vi "Save Image.vi"(8 "error in (no error)":errorcluster, 10 "Screen Shot Path":path, 11 "VISA resource name":refnum<visa-resource-name>) -> (0 "error out":errorcluster, 3 "VISA resource name out":refnum<visa-resource-name>)   [LabVIEW 2018, in "DPO4104.lvlib" / "DPO4104.lvclass"]
doc: "This VI sends the command to save a screen shot to the location specified in the input path. Tested file extensions: .png, .bmp, .tiff, .jpg, .jpeg."
uses:
  DPO4104.lvclass
  <instrlib>/Tektronix DPO MSO 2000 4000 Series/Tektronix DPO MSO 2000 4000 Series.lvlib
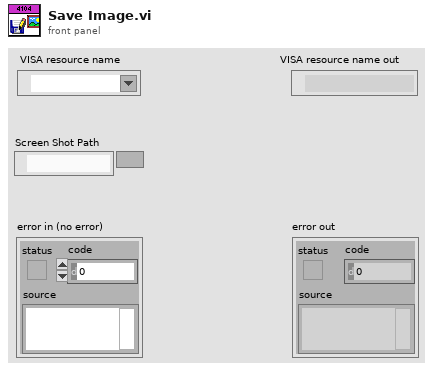
[diagram p1: front panel]
types:
  T1 = enum16{"open", "replace", "create", "open or create", "replace or create", "replace or create with confirmation"}
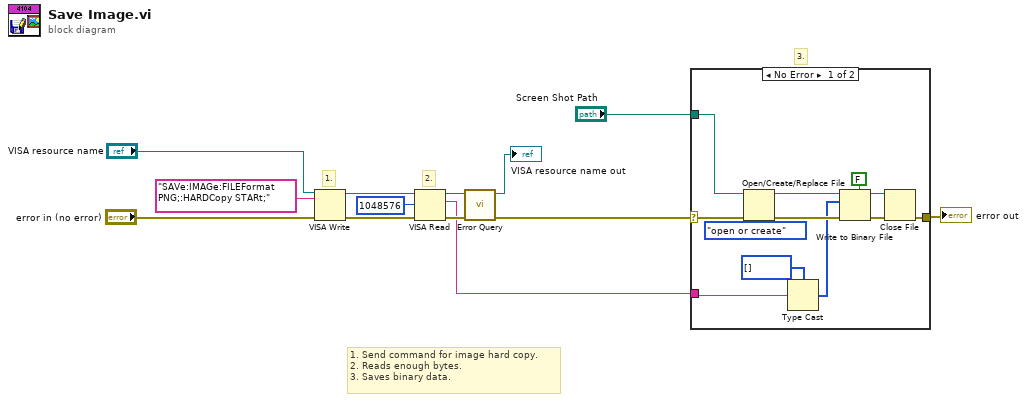
[diagram p0: block diagram]
diagram:
  # "2."
  # "1."
  # "3."
  # "1. Send command for image hard copy.\n2. Reads enough bytes.\n3. Saves binary data."
  n1 = VISA Write(VISA resource name="VISA resource name", write buffer="SAVe:IMAGe:FILEFormat PNG;:HARDCopy STARt;", error in (no error)="error in (no error)") -> (VISA resource name out=w12:refnum<visa-resource-name>, error out=w10:errorcluster)  [unwired: 1 out]
  n2 = VISA Read(VISA resource name=w12, byte count=u32 1048576, error in (no error)=w10) -> (VISA resource name out=w11:refnum<visa-resource-name>, read buffer=w5:string, error out=w9:errorcluster)  [unwired: 1 out]
  n3 = call <instrlib>:"Error Query.vi"("error in (no error)"=w9, "VISA resource name"=w11) -> ("error out"=w7:errorcluster, "VISA resource name out"=→"VISA resource name out":refnum<visa-resource-name>)  [unwired: 6 in, 2 out]
  n4 = case shown="No Error" w7 {
    selector: w7 -> [w17 w26]
    tunnel: [w16 w26] -> w6
    tunnel: w5 -> [w15 _]
    tunnel: "Screen Shot Path" -> [w14 _]
    frame No Error {
      n5 = Open/Create/Replace File(file path (use dialog)=w14, error in=w17, operation (0:open)=T1."open or create") -> (refnum out=w21:refnum<file>, error out=w23:errorcluster)  [unwired: 3 in, 1 out]
      n6 = Type Cast(type=i32[] [], x=w15) -> (*(type *) &x=w22:i32[])
      n7 = Write to Binary File(file (use dialog)=w21, data=w22, error in=w23, 5:FALSE ("prepend array or string size? (T)")) -> (refnum out=w24:refnum<file>, error out=w25:errorcluster)  [unwired: 2 in, 1 out]
      n8 = Close File(refnum=w24, error in=w25) -> (error out=w16:errorcluster)  [unwired: 1 out]
    }
    frame Error {
    }
  }
  "error out" <- w6
